vi "ReadLeftData.vi"(6 "timeout in ms (-1)":i32, 8 "error in (no error)":errorcluster, 11 "MAUI in":refnum<class "MAUI.lvclass">) -> (0 "error out":errorcluster, 2 "Left":T1, 3 "MAUI out":refnum<class "MAUI.lvclass">)   [LabVIEW 2016]
uses:
  MAUI.lvclass
  Typedefs/PanelData.ctl
  Typedefs/PanelDataNotifier.ctl
  Typedefs/PrivateEvents--MAUI.GetLeftData.ctl
  C:/Program Files (x86)/National Instruments/LabVIEW 2016/vi.lib/JKI/JKI SMO/SMO.UI/SMO.UI.lvclass
  C:/Program Files (x86)/National Instruments/LabVIEW 2016/vi.lib/JKI/JKI SMO/SMO/SMO.lvclass
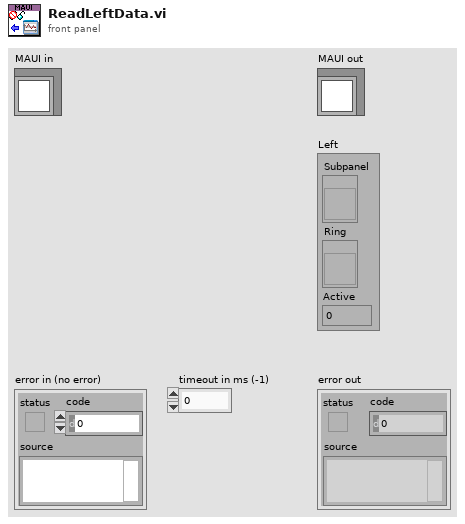
[diagram p1: front panel]
types:
  T1 = typedef "MAUI.lvclass/PanelData.ctl" = cluster{"Subpanel":refnum<vi>, "Ring":refnum<vi>, "Active":i32}
  T2 = typedef "MAUI.lvclass/PrivateEvents--MAUI.GetLeftData.ctl" = cluster{"notifier":T3}
  T3 = typedef "MAUI.lvclass/PanelDataNotifier.ctl" = refnum<notifier>
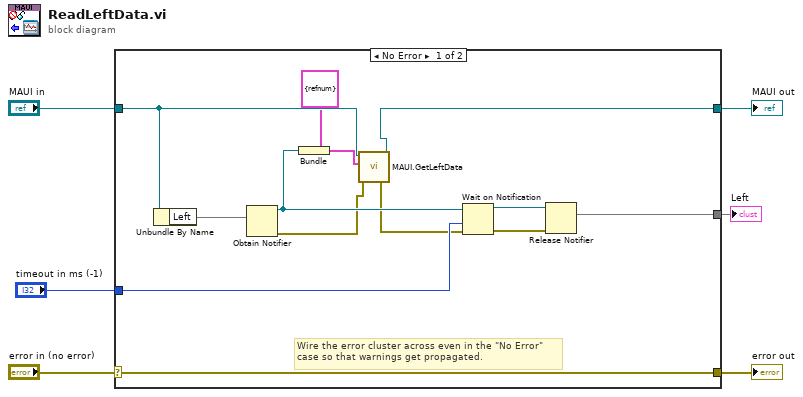
[diagram p0: block diagram]
diagram:
  n1 = case shown="No Error" "error in (no error)" {
    selector: "error in (no error)" -> [w19 w21]
    tunnel: [w19 w21] -> w3
    tunnel: [w11 w20] -> w6
    tunnel: "MAUI in" -> [w12 w20]
    tunnel: "timeout in ms (-1)" -> [w16 _]
    tunnel: [w13 _] -> w1
    frame No Error {
      # "Wire the error cluster across even in the \"No Error\"\ncase so that warnings get propagated."
      n2 = Unbundle By Name(w12) -> ("Left"=w18)
      n3 = Obtain Notifier(notification data type=w18) -> (notifier out=w17:refnum<notifier>, error out=w10:errorcluster)  [unwired: 3 in, 1 out]
      n4 = Bundle(cluster=T2 {"notifier"=refnum} ("GetLeftData"), "notifier"=w17) -> (w7:T2)
      n5 = call "MAUI.GetLeftData.vi"("error in (no error)"=w10, "GetLeftData"=w7, "MAUI"=w12) -> ("error out"=w9:errorcluster, "MAUI out"=w11:refnum<class "MAUI.lvclass">)  [unwired: 7 in]
      n6 = Wait on Notification(notifier=w17, timeout in ms (-1)=w16, error in (no error)=w9) -> (notifier out=w15:refnum<notifier>, error out=w14:errorcluster)  [unwired: 1 in, 2 out]
      n7 = Release Notifier(notifier=w15, error in (no error)=w14) -> (last notification=w13)  [unwired: 1 in, 2 out]
    }
    frame Error {
    }
  }
  "error out" <- w3
  "MAUI out" <- w6
  "Left" <- w1
